vi "daq_retroreflective_sensors.vi"(1 "Timeout":i32) -> (0 "FIFO_timeout":bool)   [LabVIEW 2018]
uses:
  <vilib>/rvi/eio/common/nirviEmuTemplateMethod_errors.vi
  <vilib>/rvi/DataTransferAndStorage/Container/Common/niFpgaContainerExecOnDevCompGetState.vi
  <vilib>/rvi/Emulation/niFpgaEmulationIsFPGAContextNoSignature.vi
  <vilib>/rvi/Emulation/niFpgaSctlEmulationGetInTimedLoop.vi
  <vilib>/rvi/errors/niFpgaSetErrorForExecOnDevCompSimple.vi
  <vilib>/rvi/eio/common/nirviEmuReportErrorAndStop.vi
  <vilib>/rvi/DataTransferAndStorage/Container/Common/niFpgaContainerGetUniqueNameForEmu.vi
  <vilib>/rvi/FIFO/Fifo_Resource/nirvififoEmulationSetSize.vi
  <vilib>/rvi/FIFO/Fifo_Resource/nirviFifoEmulationQueueMgr.vi
  <instcachedir>/0/nirviFifoEmulationQueueMgr_E5CAEC123FF24DC58D834DCA3CDAA9B5.lvgen/nirviFifoEmulationQueueMgr_E5CAEC123FF24DC58D834DCA3CDAA9B5_001.vi
  <vilib>/rvi/FIFO/Fifo_Resource/nirvififoEmulationDetermineInputValidOut.vi
  <vilib>/rvi/FIFO/Fifo_Resource/nirvififoEmulationCreateLock.vi
  <vilib>/rvi/Emulation/niFpgaProcessEmulError.vi
  <vilib>/rvi/FIFO/Fifo_Resource/nirvififoEmulationObtainLock.vi
  <vilib>/rvi/FIFO/Fifo_Resource/nirvififoEmulationReleaseLock.vi
  <vilib>/rvi/occurrence/nirviWaitOnOccurrenceBase.vi
  <vilib>/rvi/errors/nirviReportUnexpectedCaseInternalError.vi
  <vilib>/rvi/errors/nirviReportUnexpectedCaseInternalError (U32).vi
  <vilib>/Utility/error.llb/Clear Errors.vi
  <vilib>/rvi/interface/RandomDataEmulation/niFpgaRandomDataHandleErrors.vi
  <vilib>/eio/EIONode/EIONode.xnode
  <vilib>/rvi/DataTransferAndStorage/Container/XNode/niFpgaContainer.xnode
  <vilib>/rvi/FIFO/Fifo_Resource/niFpgaFifoEmulationRefIn.vi
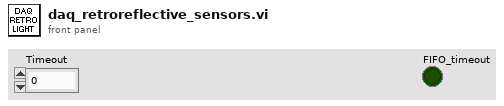
[diagram p1: front panel]
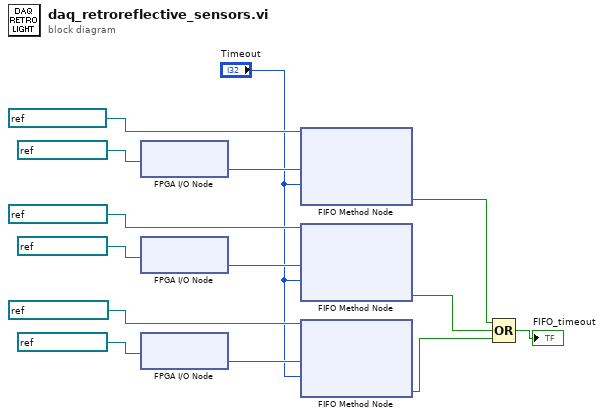
[diagram p0: block diagram]
diagram:
  n1 = xnode "FPGA I/O Node"("FPGA I/O In"=refnum<k21> "Mod2/DIO0") -> ("I/O Item"=w13:bool)  [unwired: 1 out]
  n2 = xnode "FPGA I/O Node"("FPGA I/O In"=refnum<k21> "Mod2/DIO1") -> ("I/O Item"=w10:bool)  [unwired: 1 out]
  n3 = xnode "FPGA I/O Node"("FPGA I/O In"=refnum<k21> "Mod2/DIO2") -> ("I/O Item"=w7:bool)  [unwired: 1 out]
  n4 = xnode ("FIFO Method Node")("Element"=w13, "Timeout"="Timeout", "FIFO In"=refnum<k21> "FIFO_light_FL") -> ("Timed Out?"=w4:bool)  [unwired: 1 out]
  n5 = xnode ("FIFO Method Node")("Element"=w10, "Timeout"="Timeout", "FIFO In"=refnum<k21> "FIFO_light_BL") -> ("Timed Out?"=w3:bool)  [unwired: 1 out]
  n6 = xnode ("FIFO Method Node")("Element"=w7, "Timeout"="Timeout", "FIFO In"=refnum<k21> "FIFO_light_BR") -> ("Timed Out?"=w2:bool)  [unwired: 1 out]
  n7 = Compound Arithmetic op=OR(w4, w3, w2) -> (→"FIFO_timeout":bool)
